vi "BRig_dataAnalog_valueAI0_2.vi"() -> (2 "output_valueAI0_2":i32)   [LabVIEW 2014]
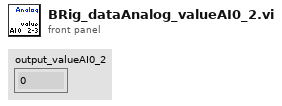
[diagram p1: front panel]
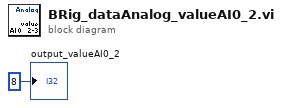
[diagram p0: block diagram]
diagram:
  "output_valueAI0_2" <- 8 ("output_iBlock")
